vi "Find Table Cell from Coordinate.vi"(8 "error in (no error)":errorcluster, 10 "Coords":T1, 11 "Table Ref":refnum<vi>) -> (0 "error out":errorcluster, 1 "Found?":bool, 2 "Column":u32, 3 "Row":u32)   [LabVIEW 2018]
uses:
  <vilib>/Utility/miscctls.llb/LVPoint32TypeDef.ctl
  <vilib>/Utility/miscctls.llb/LVRowAndColumnUnsignedTypeDef.ctl
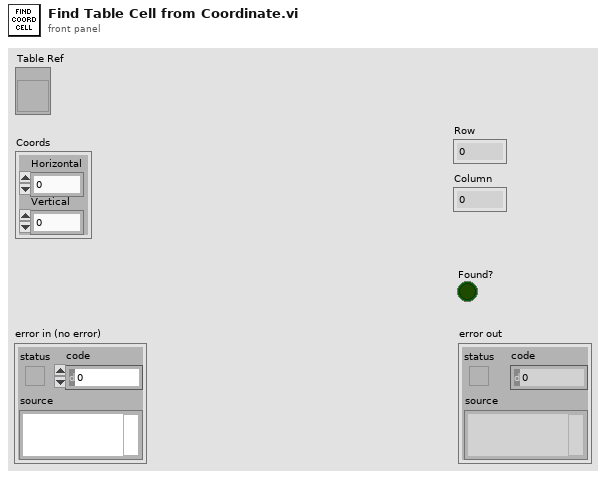
[diagram p1: front panel]
types:
  T1 = typedef "LVPoint32TypeDef.ctl" = cluster{"Horizontal":i32, "Vertical":i32}
  T2 = typedef "LVRowAndColumnUnsignedTypeDef.ctl" = cluster{"Row":u32, "Column":u32}
  T3 = typedef "LVBoundsTypeDef.ctl" = cluster{"Width":u32, "Height":u32}
  T4 = typedef "LVPositionTypeDef.ctl" = cluster{"Left":i32, "Top":i32}
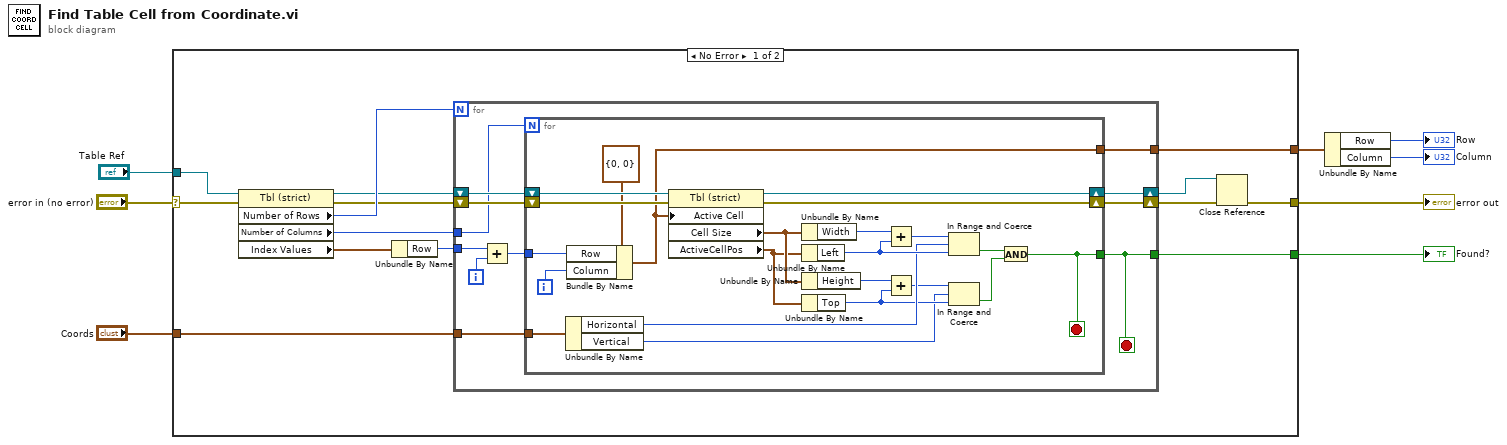
[diagram p0: block diagram]
diagram:
  n1 = case shown="No Error" "error in (no error)" {
    selector: "error in (no error)" -> [w22 w56]
    tunnel: [w10 w56] -> w7
    tunnel: "Coords" -> [w16 _]
    tunnel: [w15 _] -> w5
    tunnel: [w14 _] -> w3
    tunnel: "Table Ref" -> [w12 _]
    frame No Error {
      n2 = property class="Tbl (strict)"(reference=w12, error in=w22) -> (reference out=w19:refnum<vi>, error out=w18:errorcluster, "Number of Rows"=w21:u32, "Number of Columns"=w17:u32, "Index Values"=w13:T2)
      n3 = Unbundle By Name(w13) -> ("Row"=w20:u32)
      n4 = for {
        N: w21 -> [_]
        tunnel: w20 -> [w33]
        shift-right: [w30] -> w9
        shift-left: w19 -> [w31]
        shift-right: [w28] -> w11
        shift-left: w18 -> [w29]
        tunnel: w17 -> [w27]
        tunnel: w16 -> [w25]
        tunnel: [w24] -> w15
        tunnel: [w23] -> w14
        i -> [w32]
        stop <- w24 stop-if-true
        n5 = Add(x=w33, y=w32) -> (x+y=w26:u32)
        n6 = for {
          N: w27 -> [_]
          shift-right: [w54] -> w30
          shift-left: w31 -> [w55]
          shift-right: [w52] -> w28
          shift-left: w29 -> [w53]
          tunnel: w26 -> [w50]
          tunnel: w25 -> [w45]
          tunnel: [w35] -> w24
          tunnel: [w34] -> w23
          i -> [w49]
          stop <- w35 stop-if-true
          n7 = Unbundle By Name(w45) -> ("Horizontal"=w44:i32, "Vertical"=w38:i32)
          n8 = Bundle By Name(cluster=T2 {"Row"=0, "Column"=0} ("Index Values"), "Row"=w50, "Column"=w49) -> (w34:T2)
          n9 = property class="Tbl (strict)"(reference=w55, error in=w53, "Active Cell"=w34) -> (reference out=w54:refnum<vi>, error out=w52:errorcluster, "Cell Size"=w43:T3, "ActiveCellPos"=w42:T4)
          n10 = Unbundle By Name(w43) -> ("Width"=w48:u32)
          n11 = Unbundle By Name(w42) -> ("Left"=w47:i32)
          n12 = Unbundle By Name(w43) -> ("Height"=w41:u32)
          n13 = Unbundle By Name(w42) -> ("Top"=w39:i32)
          n14 = Add(x=w48, y=w47) -> (x+y=w46:u32)
          n15 = Add(x=w41, y=w39) -> (x+y=w40:u32)
          n16 = In Range and Coerce(upper limit=w46, x=w44, lower limit=w47) -> (In Range?=w37:bool)  [unwired: 1 out]
          n17 = In Range and Coerce(upper limit=w40, x=w38, lower limit=w39) -> (In Range?=w36:bool)  [unwired: 1 out]
          n18 = And(x=w37, y=w36) -> (x .and. y?=w35:bool)
        }
      }
      n19 = Close Reference(reference=w9, error in (no error)=w11) -> (error out=w10:errorcluster)
    }
    frame Error {
    }
  }
  "error out" <- w7
  "Found?" <- w5
  n20 = Unbundle By Name(w3) -> ("Row"=→"Row":u32, "Column"=→"Column":u32)
